vi "Get Resource ID.vi"(11 "AnalogIn in":refnum<class "AnalogIn.lvclass">) -> (2 "Resource ID":string)   [LabVIEW 2020, in "CTI.lvlib" / "AnalogIn.lvclass"]
uses:
  AnalogIn.lvclass
  AnalogIn.lvclass/AnalogIn.ctl
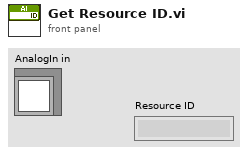
[diagram p1: front panel]
types:
  T1 = typedef "CTI.lvlib/ADC Number.ctl" = i8
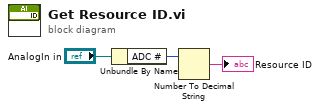
[diagram p0: block diagram]
diagram:
  n1 = Unbundle By Name("AnalogIn in") -> ("ADC #"=w2:T1)
  n2 = Number To Decimal String(number=w2) -> (decimal integer string=→"Resource ID":string)  [unwired: 1 in]
